vi "_Parse Detected Allocation Segment.vi"(8 "error in (no error)":errorcluster, 10 "Input String":string, 11 "VISA resource name":refnum<visa-resource-name>) -> (0 "error out":errorcluster, 1 "Detected Allocation":T2, 2 "Reliability Results":T1, 3 "VISA resource name out":refnum<visa-resource-name>)   [LabVIEW 2020, in "Rohde&Schwarz CMXP NR FR2 Measurement.lvlib"]
uses:
  <instrlib>/Rohde&Schwarz CMXP NR FR2 Measurement/Rohde&Schwarz CMXP NR FR2 Measurement.lvlib
  <instrlib>/Rohde&Schwarz CMXP NR FR2 Measurement/Private/rsidr_core.llb/rsidr_core.lvlib
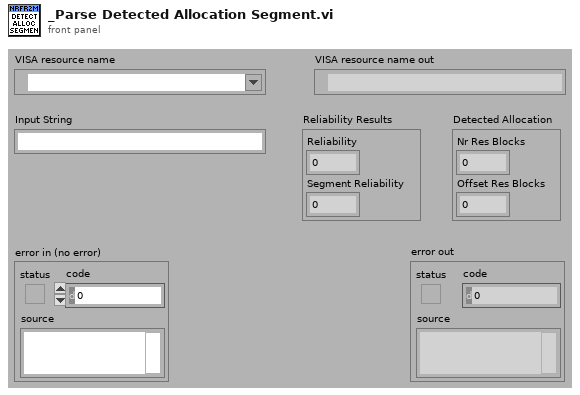
[diagram p1: front panel]
types:
  T1 = cluster{"Reliability":i32, "Segment Reliability":i32}
  T2 = cluster{"Nr Res Blocks":i32, "Offset Res Blocks":i32}
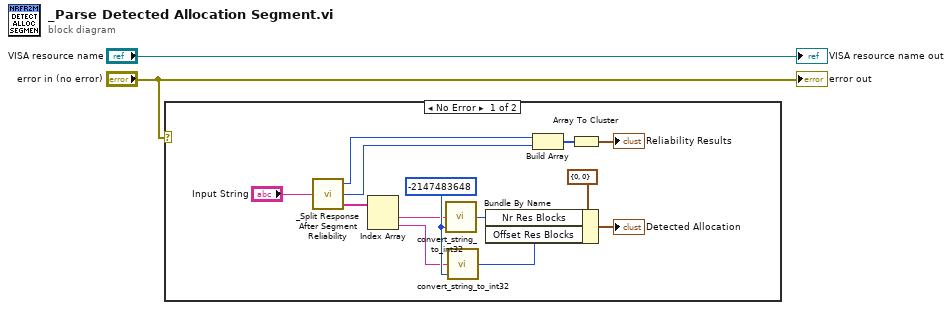
[diagram p0: block diagram]
diagram:
  n1 = case shown="No Error" "error in (no error)" {
    frame No Error {
      w15 = -2147483648
      n2 = call <instrlib>:"_Split Response After Segment Reliability.vi"("Input String"="Input String") -> ("Response out"=w10:string[], "Segment Reliability"=w5:i32, "Reliability"=w6:i32)
      n3 = Index Array(array=w10) -> (element #1=w8:string, element #2=w7:string)  [unwired: 2 in]
      n4 = call <instrlib>:"convert_string_to_int32.vi"("default (0)"=w15, "String in"=w8) -> ("int32 value out"=w12:i32)  [unwired: 3 in]
      n5 = call <instrlib>:"convert_string_to_int32.vi"("default (0)"=w15, "String in"=w7) -> ("int32 value out"=w11:i32)  [unwired: 3 in]
      n6 = Bundle By Name(cluster=T2 {"Nr Res Blocks"=0, "Offset Res Blocks"=0} ("Detected Allocation"), "Nr Res Blocks"=w12, "Offset Res Blocks"=w11) -> (→"Detected Allocation":T2)
      n7 = Build Array(w6, w5) -> (w4:i32[])
      n8 = Array To Cluster(array=w4) -> (cluster=→"Reliability Results":cluster{"[0]":i32, "[1]":i32})
    }
    frame Error {
    }
  }
  "VISA resource name out" <- "VISA resource name"
  "error out" <- "error in (no error)"
